vi "Refresh Rooms Status.vi"(0 "Rooms Manager UI in":refnum<class "Rooms Manager UI.lvclass">, 5 "Room Details":T1[](array[typedef]), 11 "error in (no error)":errorcluster) -> (4 "Rooms Manager UI out":refnum<class "Rooms Manager UI.lvclass">, 15 "error out":errorcluster)   [LabVIEW 2023, in "Rooms Manager UI.lvlib" / "Rooms Manager UI.lvclass"]
uses:
  Rooms Manager UI.lvclass
  Room Status.ctl
  Rooms Manager UI.lvclass/Rooms Manager UI.ctl
  Utilities/Utilities.lvlib
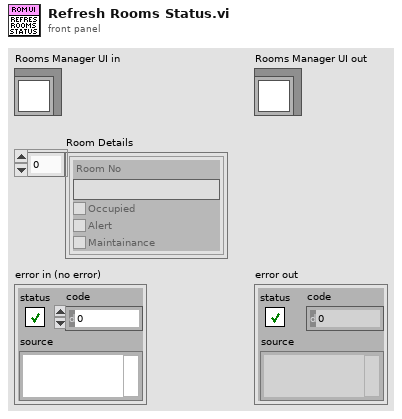
[diagram p1: front panel]
types:
  T1 = typedef "Rooms Manager UI.lvlib/Rooms Manager UI.lvclass/Room Status.ctl" = cluster{"Room No":string, "Occupied":bool, "Alert":bool, "Maintainance":bool}
  T2 = cluster{"Room No":string, "Alert":bool, "Occupied":bool, "Maintainance":bool, "IsActive":bool}[][]
  T3 = cluster{"Room No":string, "Alert":bool, "Occupied":bool, "Maintainance":bool, "IsActive":bool}[]
  T4 = cluster{"Room No":string, "Alert":bool, "Occupied":bool, "Maintainance":bool, "IsActive":bool}
  T5 = enum8{"Enabled", "Disabled", "Disabled and Grayed Out"}
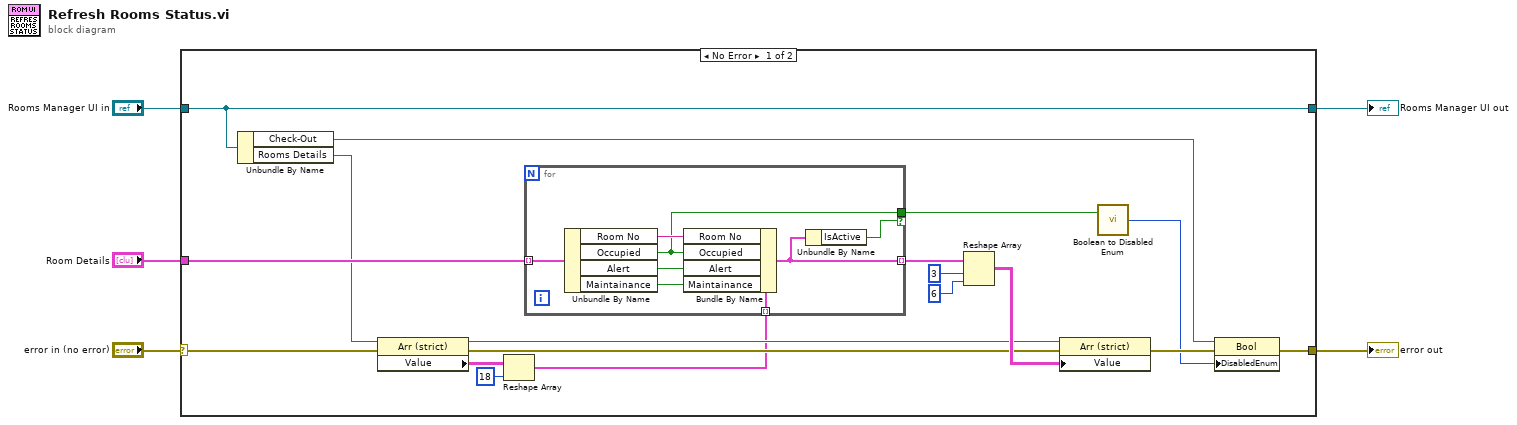
[diagram p0: block diagram]
diagram:
  n1 = case shown="No Error" "error in (no error)" {
    selector: "error in (no error)" -> [w13 w33]
    tunnel: [w9 w33] -> w4
    tunnel: [w23 w32] -> w2
    tunnel: "Rooms Manager UI in" -> [w23 w32]
    tunnel: "Room Details" -> [w21 _]
    frame No Error {
      n2 = Unbundle By Name(w23) -> ("Check-Out"=w8:refnum<vi>, "Rooms Details"=w16:refnum<vi>)
      n3 = property class="Arr (strict)"(reference=w16, error in=w13) -> (reference out=w15:refnum<vi>, error out=w14:errorcluster, "Value"=w12:T2)
      n4 = Reshape Array(w12, 18 ("dimension size")) -> (w10:T3)
      n5 = for {
        tunnel: w21 -> [w31] mode=indexing
        tunnel: [w26] -> w20 mode=indexing
        tunnel: w10 -> [w27] mode=indexing
        tunnel: [w25] -> w6 if=w24
        n6 = Unbundle By Name(w31) -> ("Room No"=w30:string, "Occupied"=w25:bool, "Alert"=w29:bool, "Maintainance"=w28:bool)
        n7 = Bundle By Name(cluster=w27, "Room No"=w30, "Occupied"=w25, "Alert"=w29, "Maintainance"=w28) -> (w26:T4)
        n8 = Unbundle By Name(w26) -> ("IsActive"=w24:bool)
      }
      n9 = Reshape Array(w20, 3 ("dimension size"), 6 ("dimension size")) -> (w19:T2)
      n10 = property class="Arr (strict)"(reference=w15, error in=w14, "Value"=w19) -> (error out=w22:errorcluster)  [unwired: 1 out]
      n11 = call "Boolean to Disabled Enum.vi"("Enable"=w6) -> ("Disabled"=w7:T5)  [unwired: 1 in]
      n12 = property class="Bool"(reference=w8, error in=w22, "DisabledEnum"=w7) -> (error out=w9:errorcluster)  [unwired: 1 out]
    }
    frame Error {
    }
  }
  "error out" <- w4
  "Rooms Manager UI out" <- w2
